vi "pressures.vi"() -> ()   [LabVIEW 2018]
panel:
  out "Chamber (mbar)":dbl format="%#_3e"
  out "Back (mbar)":dbl format="%#_3e"
  in  "stop":bool
  # "Turbo Pump"
  # "Scroll (Roughing) Pump"
  # "Pump"
  # "Back\nPressure\nReadout"
  # "Gate"
  # "Roughing"
  # "Chamber\nPressure\nReadout"
  # "Chamber"
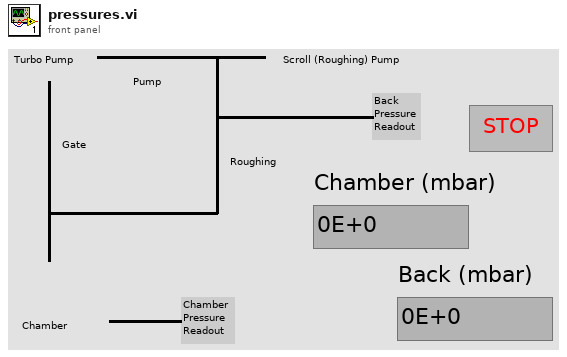
[diagram p1: front panel]
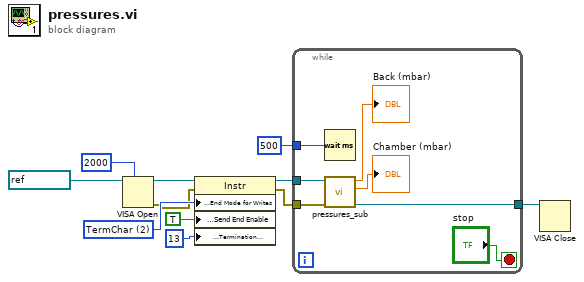
[diagram p0: block diagram]
diagram:
  w11 = u16 2 items=["None", "Last Bit", "TermChar", "Break"] ("Serial Settings:End Mode for Writes")
  n1 = VISA Open(timeout (0)=u32 2000 ("VISA Open timeout (0)"), VISA resource name=refnum<visa-resource-name> "COM7") -> (VISA resource name=w4:refnum<visa-resource-name>, error out=w1:errorcluster)  [unwired: 3 in]
  n2 = property class="Instr"(reference=w4, error in=w1, "Serial Settings:End Mode for Writes"=w11, "Message Based Settings:Send End Enable"=TRUE, "Message Based Settings:Termination Character"=u8 13) -> (reference out=w8:refnum<visa-resource-name>, error out=w2:errorcluster)
  n3 = while {
    tunnel: w8 -> [w16]
    tunnel: [w13] -> w7
    tunnel: u32 500 ("milliseconds to wait") -> [w17]
    tunnel: w2 -> [w12]
    stop <- "stop" stop-if-true
    n4 = Wait (ms)(milliseconds to wait=w17) -> ()  [unwired: 1 out]
    n5 = call "pressures_sub.vi"("error in (no error)"=w12, "VISA Session In"=w16) -> ("VISA Session (Dup) Gauge1"=w13:refnum<visa-resource-name>, "Chamber (mbar)"=→"Chamber (mbar)":dbl, "Back (mbar)"=→"Back (mbar)":dbl)  [unwired: 7 in]
  }
  n6 = VISA Close(VISA resource name=w7) -> ()  [unwired: 1 in, 1 out]
